vi "SeperateLayersPython.vi"(8 "error in (no error)":errorcluster, 10 "Py Session":refnum<k35>, 11 "Cluster":T1) -> (0 "error out":errorcluster, 2 "Py Session out":refnum<k35>, 3 "return value":cluster{"Success":bool, "Status":string})   [LabVIEW 2022 SP3, in "DLP2.lvclass"]
uses:
  DLP2.lvclass
  DataTypes/SeperateLayersPython--cluster.ctl
  Common/Controls/PythonVersion--Enum.ctl
  DLP2.lvclass/DLP2.ctl
panel:
  out "Sys Exec Command":string
  out "targetMaterials":string[](array[string])
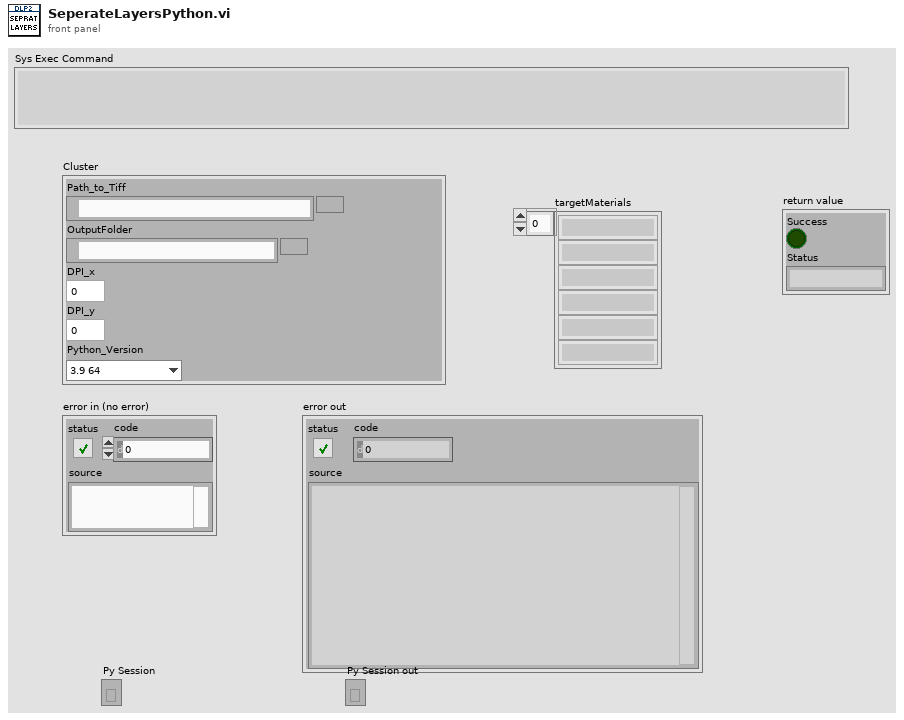
[diagram p1: front panel]
types:
  T1 = typedef "SeperateLayersPython--cluster.ctl" = cluster{"Path_to_Tiff":path, "OutputFolder":path, "DPI_x":i32, "DPI_y":i32, "Python_Version":T2}
  T2 = typedef "PythonVersion--Enum.ctl" = enum16{"3.9 64", "3.9 32", "3.12 64", "3.12 32"}
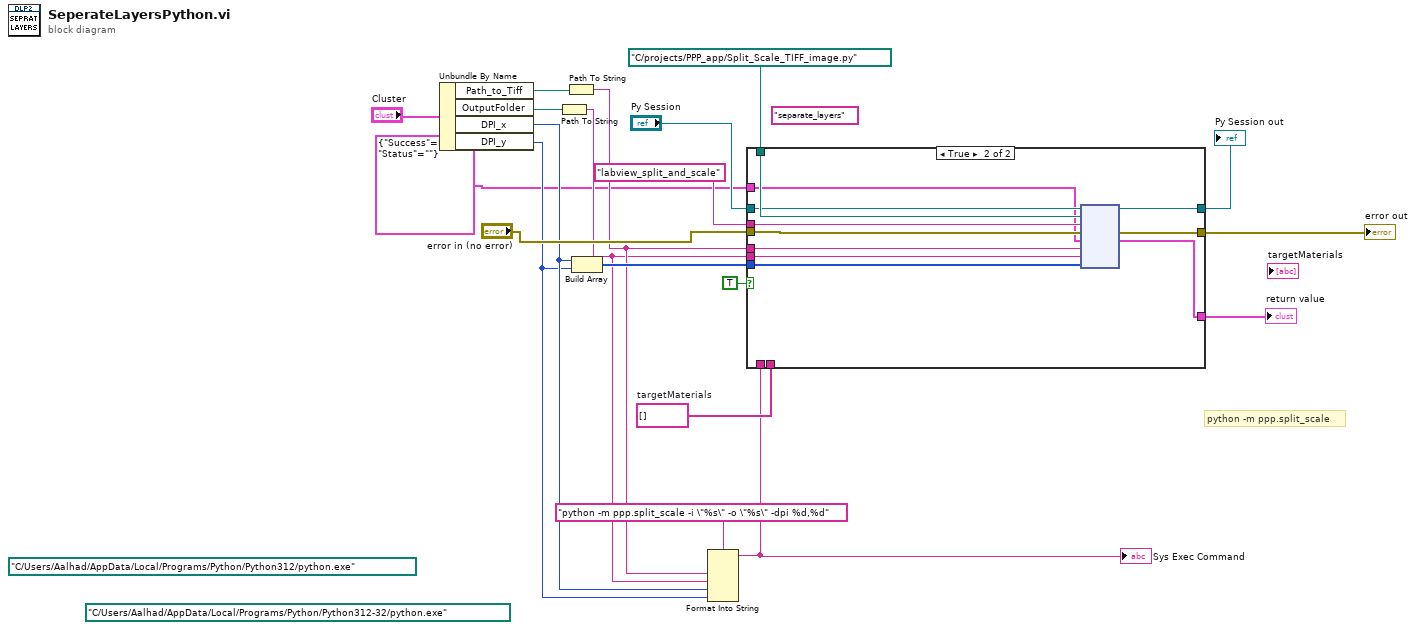
[diagram p0: block diagram]
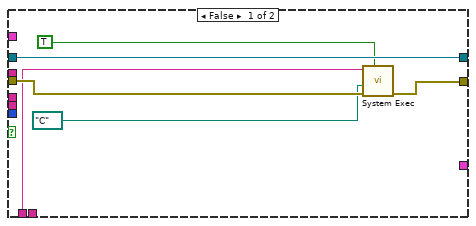
[diagram p2: hidden frame]
diagram:
  (unwired) "separate_layers" ("function name")
  (unwired) path "C:/Users/Aalhad/AppData/Local/Programs/Python/Python312-32/python.exe" ("Python path")
  (unwired) path "C:/Users/Aalhad/AppData/Local/Programs/Python/Python312/python.exe" ("Python path")
  w10 = string[] []  # targetMaterials
  # "python -m ppp.split_scale"
  n1 = Unbundle By Name("Cluster") -> ("Path_to_Tiff"=w16:path, "OutputFolder"=w15:path, "DPI_x"=w4:i32, "DPI_y"=w3:i32)
  n2 = Path To String(path=w15) -> (string=w5:string)
  n3 = Path To String(path=w16) -> (string=w6:string)
  n4 = Build Array(w4, w3) -> (w14:i32[])
  n5 = Format Into String(format string="python -m ppp.split_scale -i \"%s\" -o \"%s\" -dpi %d,%d", w6, w5, w4, w3) -> (resulting string=w7:string)  [unwired: 2 in, 1 out]
  "Sys Exec Command" <- w7
  n6 = case shown="True" TRUE {
    tunnel: "labview_split_and_scale" ("function name") -> [_ w37]
    tunnel: [w26 w36] -> w19
    tunnel: path "C:/projects/PPP_app/Split_Scale_TIFF_image.py" -> [_ w35]
    tunnel: w6 -> [_ w34]
    tunnel: w5 -> [_ w33]
    tunnel: w14 -> [_ w32]
    tunnel: "Py Session" -> [w26 w31]
    tunnel: "error in (no error)" -> [w24 w30]
    tunnel: [w23 w29] -> w11
    tunnel: w10 -> [_ _]
    tunnel: w7 -> [w21 _]
    tunnel: cluster{"Success":bool, "Status":string} {"Success"=FALSE, "Status"=""} -> [_ w28]
    tunnel: [_ w27] -> w1
    frame False {
      n7 = call <vilib>:"System Exec.vi"("wait until completion? (T)"=TRUE, "error in (no error)"=w24, "working directory"=path "C:/", "command line"=w21) -> ("error out"=w23:errorcluster)  [unwired: 4 in, 3 out]
    }
    frame True {
      n8 = node(w31, w35, w37, w30, w28, w34, w33, w32) -> (w36:refnum<k35>, w29:errorcluster, w27:cluster{"Success":bool, "Status":string})  [unwired: 3 in, 2 out]
    }
  }
  "error out" <- w11
  "Py Session out" <- w19
  "return value" <- w1
